vi "Read Sub Panel Turnos 1.vi"(8 "error in (no error)":errorcluster, 11 "Turnos in":refnum<class "Turnos.lvclass">) -> (0 "error out":errorcluster, 2 "Sub Panel Turnos":refnum<vi>, 3 "Turnos out":refnum<class "Turnos.lvclass">)   [LabVIEW 2020, in "Turnos.lvlib" / "Turnos.lvclass"]
uses:
  Turnos.lvclass
  Turnos.lvclass/Turnos.ctl
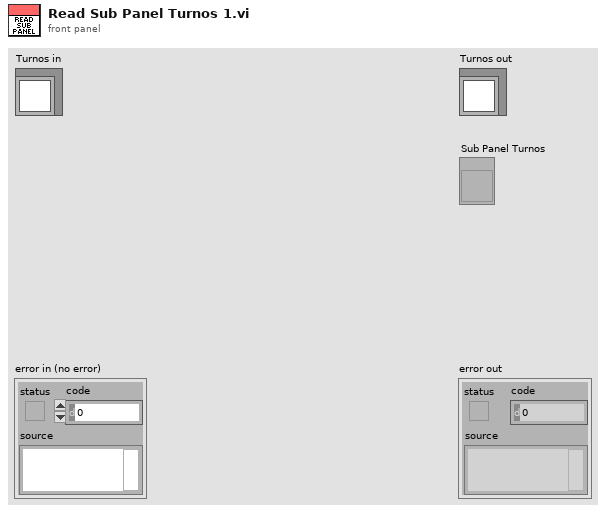
[diagram p1: front panel]
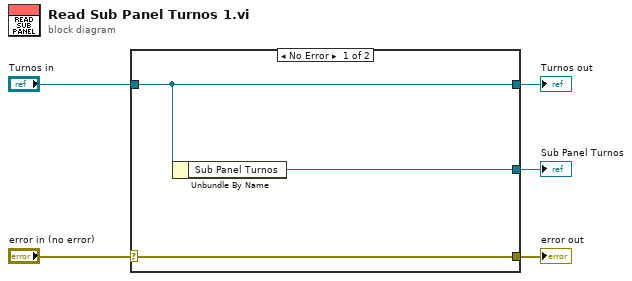
[diagram p0: block diagram]
diagram:
  n1 = case shown="No Error" "error in (no error)" {
    selector: "error in (no error)" -> [w8 w9]
    tunnel: [w8 w9] -> w4
    tunnel: [w7 w10] -> w2
    tunnel: "Turnos in" -> [w7 w10]
    tunnel: [w6 _] -> w1
    frame No Error {
      n2 = Unbundle By Name(w7) -> ("Sub Panel Turnos"=w6:refnum<vi>)
    }
    frame Error {
    }
  }
  "error out" <- w4
  "Turnos out" <- w2
  "Sub Panel Turnos" <- w1
